vi "Destroy.vi"(11 "Base Queue in":refnum<class "Base Queue.lvclass">) -> (3 "Base Queue out":refnum<class "Base Queue.lvclass">)   [LabVIEW 2021, in "jettl.lvlib" / "Base Queue.lvlib" / "Base Queue.lvclass"]
uses:
  Base Queue.lvclass
  Base Queue.lvclass/Base Queue.ctl
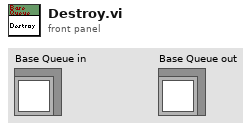
[diagram p1: front panel]
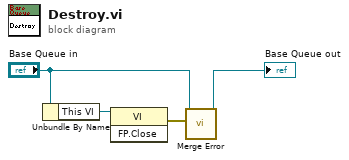
[diagram p0: block diagram]
diagram:
  n1 = Unbundle By Name("Base Queue in") -> ("This VI"=w4:refnum<vi>)
  n2 = invoke class="VI" method="FP.Close"(reference=w4) -> (error out=w3:errorcluster)  [unwired: 2 in, 2 out]
  n3 = call-dynamic "Merge Error.vi"("Error"=w3, "Base Queue in"="Base Queue in") -> ("Base Queue out"=→"Base Queue out":refnum<class "Base Queue.lvclass">)  [unwired: 9 in]
